vi "Binary Number to Decimal Number_LV2012_NI Verified.vi"(11 "Binary number":i32=422 format="%.0b") -> (3 "Decimal number":i64)   [LabVIEW 2017]
doc: "This VI converts a binary number into the correct numeric representation"
panel:
  # "Overview: This VI allows you to convert a binary number into the correct numeric representation\nRequirements: LabVIEW 2012(or compatible)\nInstructions:\n1. Enter the binary number\n2. Run the VI"
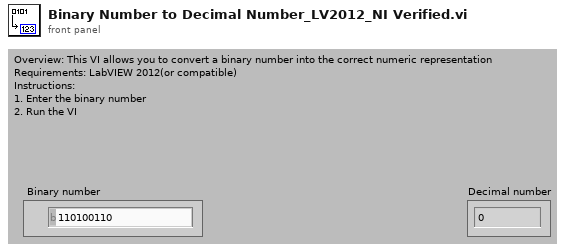
[diagram p1: front panel]
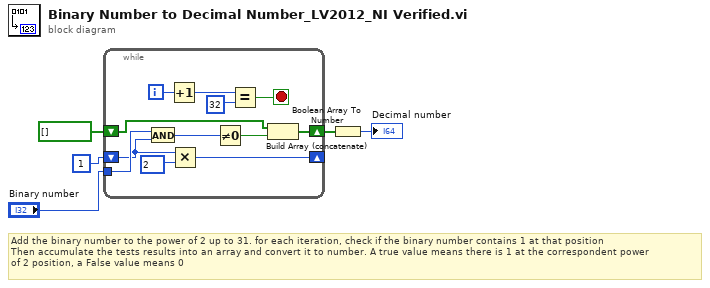
[diagram p0: block diagram]
diagram:
  # "Add the binary number to the power of 2 up to 31. for each iteration, check if the binary number contains 1 at that position\nThen accumulate the tests results into an array and convert it to number. A true value means there is 1 at the correspondent power \nof 2 position, a False value means 0"
  n1 = while {
    tunnel: "Binary number" -> [w14]
    shift-right: [w11] -> _
    shift-left: 1 ("x") -> [w13]
    shift-right: [w8] -> w3
    shift-left: bool[] [] -> [w7]
    i -> [w9]
    stop <- w17 stop-if-true
    n2 = And(x=w14, y=w13) -> (x .and. y?=w10:i32)
    n3 = Increment(x=w9) -> (x+1=w16:i32)
    n4 = Multiply(x=w13, y=2) -> (x*y=w11:i32)
    n5 = Not Equal To 0?(x=w10) -> (x != 0?=w6:bool)
    n6 = Equal?(x=w16, y=32) -> (x = y?=w17:bool)
    n7 = Build Array (concatenate)(w7, w6) -> (w8:bool[])
  }
  n8 = Boolean Array To Number(Boolean array=w3) -> (number=→"Decimal number":u32)
